vi "Calculate dts from Timestamps.vi"(4 "TimeStamps":u64[](array[numeric])) -> (1 "dts":u64[](array[numeric]))   [LabVIEW 2020]
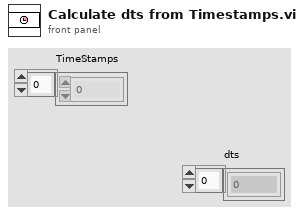
[diagram p1: front panel]
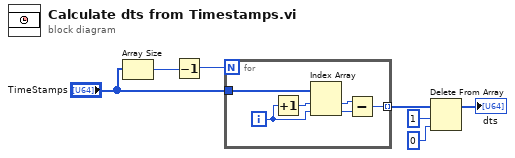
[diagram p0: block diagram]
diagram:
  n1 = Array Size(array="TimeStamps") -> (size(s)=w1:i32)
  n2 = Decrement(x=w1) -> (x-1=w2:i32)
  n3 = for {
    N: w2 -> [_]
    tunnel: "TimeStamps" -> [w13]
    tunnel: [w10] -> w4 mode=indexing
    i -> [w8]
    n4 = Increment(x=w8) -> (x+1=w9:i32)
    n5 = Index Array(array=w13, index #1=w9, index #2=w8) -> (element #1=w12:u64, element #2=w11:u64)
    n6 = Subtract(x=w12, y=w11) -> (x-y=w10:u64)
  }
  n7 = Delete From Array(array=w4, length=1, index=0) -> (array with subset deleted=→"dts":u64[])  [unwired: 1 out]
